vi "Error - Check Error.vi"(8 "error in (no error)":errorcluster, 11 "View Model":T2) -> (0 "error out":errorcluster, 3 "View Model":T2)   [LabVIEW 2017]
uses:
  View Model/Controls/View Model.ctl
  Controls/Error Model.ctl
  Controls/Error Type.ctl
  View Model/Controls/Shared Model.ctl
panel:
  in  "Error Type":T1
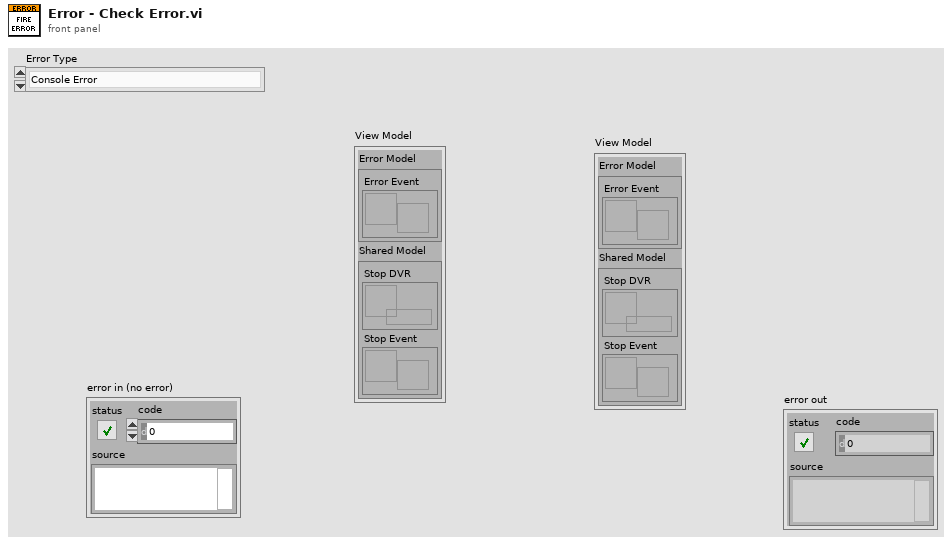
[diagram p1: front panel]
types:
  T1 = typedef "Error Type.ctl" = enum16{"Console Error", "Process Step Error", "Sensor Interface IO Error"}
  T2 = typedef "View Model.ctl" = cluster{"Error Model":T3, "Shared Model":T4}
  T3 = typedef "Error Model.ctl" = cluster{"Error Event":refnum<user-event>}
  T4 = typedef "Shared Model.ctl" = cluster{"Stop DVR":refnum<data-value>, "Stop Event":refnum<user-event>}
  T5 = cluster{"Error Type":T1, "error in (no error)":errorcluster}
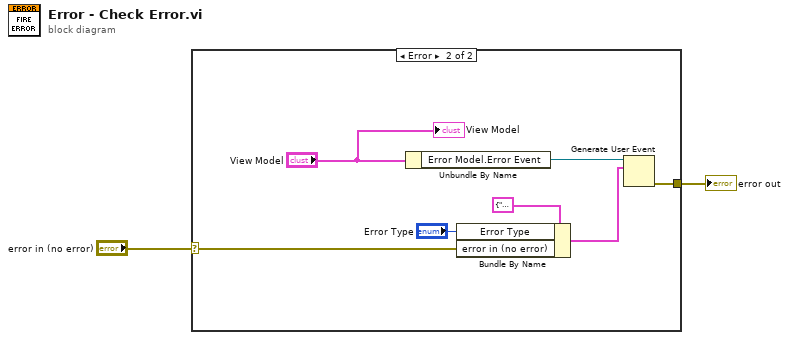
[diagram p0: block diagram]
diagram:
  n1 = case shown="Error" "error in (no error)" {
    selector: "error in (no error)" -> [w3 w4]
    tunnel: [w3 w5] -> w2
    frame No Error {
    }
    frame Error {
      n2 = Unbundle By Name("View Model") -> ("Error Model.Error Event"=w10:refnum<user-event>)
      n3 = Bundle By Name(cluster=T5 {"Error Type"=enum."Console Error", "error in (no error)"={"status"=FALSE, "code"=0, "source"=""}} ("event data"), "Error Type"="Error Type", "error in (no error)"=w4) -> (w7:T5)
      n4 = Generate User Event(user event=w10, event data cluster=w7) -> (error out=w5:errorcluster)  [unwired: 2 in, 1 out]
      "View Model" <- "View Model"
    }
  }
  "error out" <- w2
